vi "GameSettings.vi"(8 "error in (no error)":errorcluster, 11 "main Data in":T3) -> (0 "error out":errorcluster, 3 "main Data out":T3)   [LabVIEW 2020]
uses:
  TypeDef/main-data.ctl
  TypeDef/board-type.ctl
  TypeDef/display-trunct.ctl
  TypeDef/tiles-trunct.ctl
  TypeDef/tiles-key-trunct.ctl
panel:
  in  "Time between steps (ms)":u32
  out "Display-trunct":T1
  in  "OK Button":bool
  in  "Cancel Button":bool
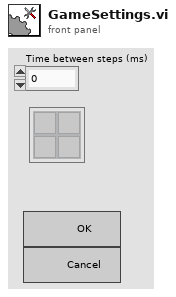
[diagram p1: front panel]
types:
  T1 = typedef "display-trunct.ctl" = T2[][]
  T2 = typedef "tiles-trunct.ctl" = u16
  T3 = typedef "main-data.ctl" = cluster{"Board Type":T4, "Size":i32, "Board":T1, "Interval (ms)":i32}
  T4 = typedef "board-type.ctl" = enum16{"Open", "Walled", "Custom"}
  T5 = typedef "tiles-key-trunct.ctl" = enum16{"ground", "wall", "head (right)", "head (up)", "head (left)", "head (down)", "L-turn (right-up)", "L-turn (up-left)", "L-turn (left-down)", "L-turn (down-right)", "body (right)", "body (up)", "body (left)", "body (down)", "R-turn (right-down)", "R-turn (up-right)", "R-turn (left-up)", "R-turn (down-left)", "tail (right)", "tail (up)", "tail (left)", "tail (down)"}
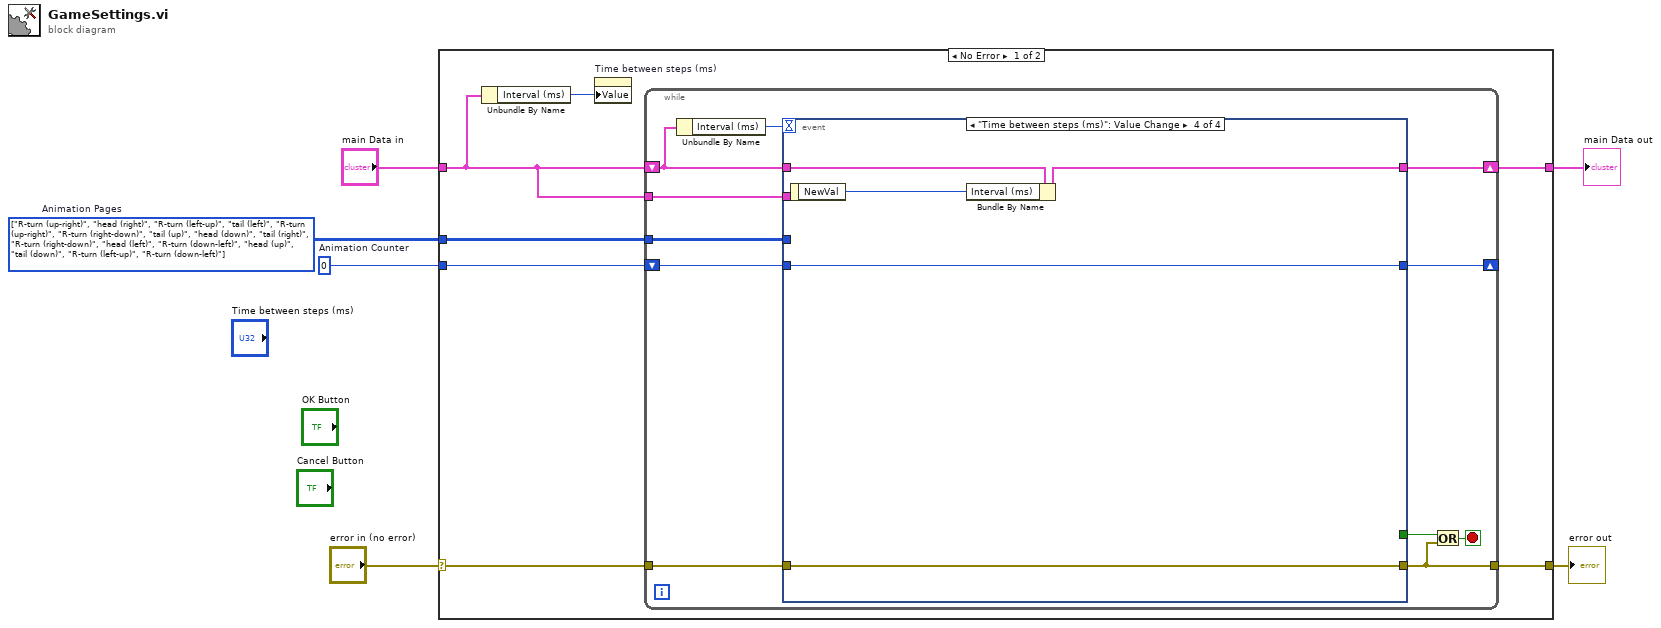
[diagram p0: block diagram]
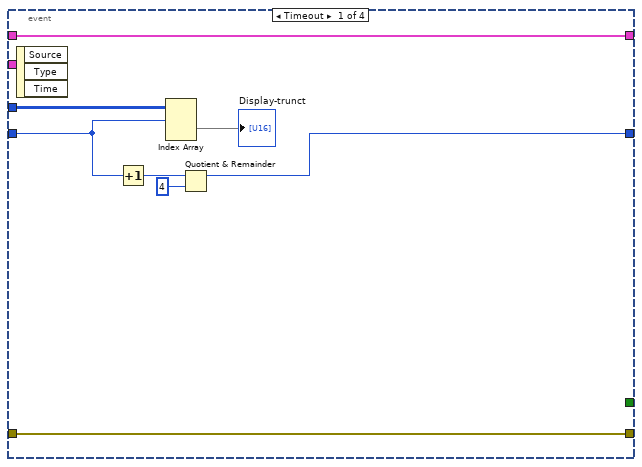
[diagram p2: hidden frame]
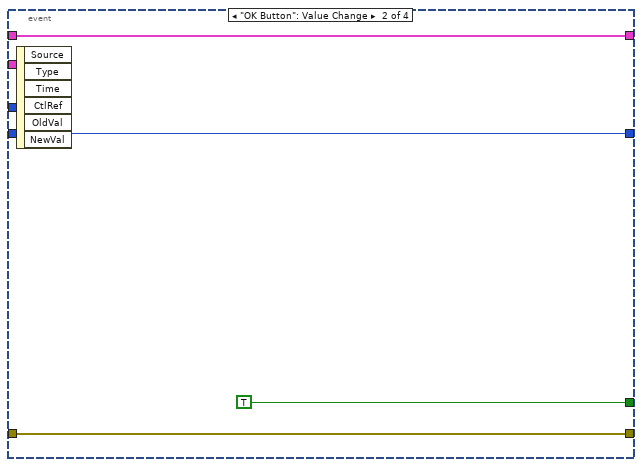
[diagram p3: hidden frame]
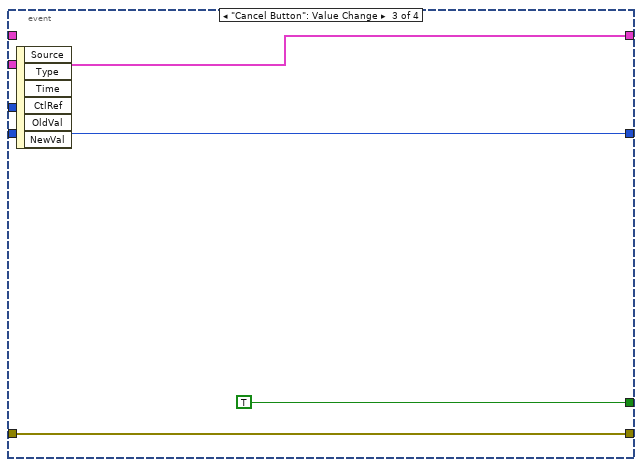
[diagram p4: hidden frame]
diagram:
  w1 = 0  # Animation Counter
  w2 = T5[][][] [[[enum."R-turn (up-right)", enum."head (right)"], [enum."R-turn (left-up)", enum."tail (left)"]], [[enum."R-turn (up-right)", enum."R-turn (right-down)"], [enum."tail (up)", enum."head (down)"]], [[enum."tail (right)", enum."R-turn (right-down)"], [enum."head (left)", enum."R-turn (down-left)"]], [[enum."head (up)", enum."tail (down)"], [enum."R-turn (left-up)", enum."R-turn (down-left)"]]] items=["ground", "wall", "head (right)", "head (up)", "head (left)", "head (down)", "L-turn (right-up)", "L-turn (up-left)", "L-turn (left-down)", "L-turn (down-right)", "body (right)", "body (up)", "body (left)", "body (down)", "R-turn (right-down)", "R-turn (up-right)", "R-turn (left-up)", "R-turn (down-left)", "tail (right)", "tail (up)", "tail (left)", "tail (down)"]  # Animation Pages
  n1 = case shown="No Error" "error in (no error)" {
    selector: "error in (no error)" -> [w13 w47]
    tunnel: [w12 w47] -> w5
    tunnel: "main Data in" -> [w8 w46]
    tunnel: [w11 w46] -> w3
    tunnel: w2 -> [w10 _]
    tunnel: w1 -> [w9 _]
    frame No Error {
      n2 = Unbundle By Name(w8) -> ("Interval (ms)"=w7:i32)
      n3 = property on="Time between steps (ms)" class="DigNum (strict)"("Value"=w7) -> ()  [unwired: 2 in, 2 out]
      n4 = while {
        tunnel: w13 -> [w24]
        tunnel: [w19] -> w12
        tunnel: w8 -> [w17]
        shift-right: [w22] -> w11
        shift-left: w8 -> [w21]
        shift-right: [w14] -> _
        shift-left: w9 -> [w15]
        tunnel: w10 -> [w16]
        stop <- w20 stop-if-true
        n5 = Unbundle By Name(w21) -> ("Interval (ms)"=w23:i32)
        n6 = event shown="[3] \"Time between steps (ms)\": Value Change" {
          selector: _ -> [_ _ _ _]
          dyn-events: _ -> [_ _ _ _]
          timeout: w23 -> [_ _ _ _]
          tunnel: [w32 w36 w40 w41] -> w19
          tunnel: w24 -> [w32 w36 w40 w41]
          tunnel: w21 -> [w31 w35 _ w44]
          tunnel: [w31 w35 w38 w43] -> w22
          tunnel: [_ TRUE TRUE _] -> w18
          tunnel: w17 -> [_ _ w38 _]
          tunnel: w16 -> [w30 _ _ _]
          tunnel: w15 -> [w28 w33 w37 w45]
          tunnel: [w25 w33 w37 w45] -> w14
          event Timeout {
            n7 = event-data() -> ()  [unwired: 1 in, 3 out]
            n8 = Increment(x=w28) -> (x+1=w27:i32)
            n9 = Index Array(array=w30, index (dim 0)=w28) -> (element=→"Display-trunct":T5[][])  [unwired: 2 in]
            n10 = Quotient & Remainder(x=w27, y=4) -> (x-y*floor(x/y)=w25:i32)  [unwired: 1 out]
          }
          event "OK Button": Value Change {
            n11 = event-data() -> ()  [unwired: 1 in, 6 out]
          }
          event "Cancel Button": Value Change {
            n12 = event-data() -> ()  [unwired: 1 in, 6 out]
          }
          event "Time between steps (ms)": Value Change {
            n13 = event-data() -> ("NewVal"=w42:u32)  [unwired: 1 in]
            n14 = Bundle By Name(cluster=w44, "Interval (ms)"=w42) -> (w43:T3)
          }
        }
        n15 = Or(x=w18, y=w19) -> (x .or. y?=w20:bool)
      }
    }
    frame Error {
    }
  }
  "error out" <- w5
  "main Data out" <- w3
